vi "CCSA RPJ SLJC PF SubVI009.vi"(2 "Patrón original":T1, 3 "Toma original":T1) -> (0 "Toma original":T1(plugin-control), 1 "Patrón corregido":T1(plugin-control))   [LabVIEW 2021]
doc: "Traslada el patrón a la misma posición que la toma de la cámara para empalmar sus contornos"
uses:
  <vilib>/vision/Image Controls.llb/IMAQ Image.ctl
panel:
  out "Patrón original":T1(plugin-control)
  out "Centroide Patron":cluster{"X Centroid":sgl, "Y Centroid":sgl}
  out "Centroide Captura":cluster{"X Centroid":sgl, "Y Centroid":sgl}
  # "CUEVAS CERÓN SERGIO ALBERTO\nREYES PÉREZ JAVIER\nSALCEDO LICEA JUAN CARLOS"
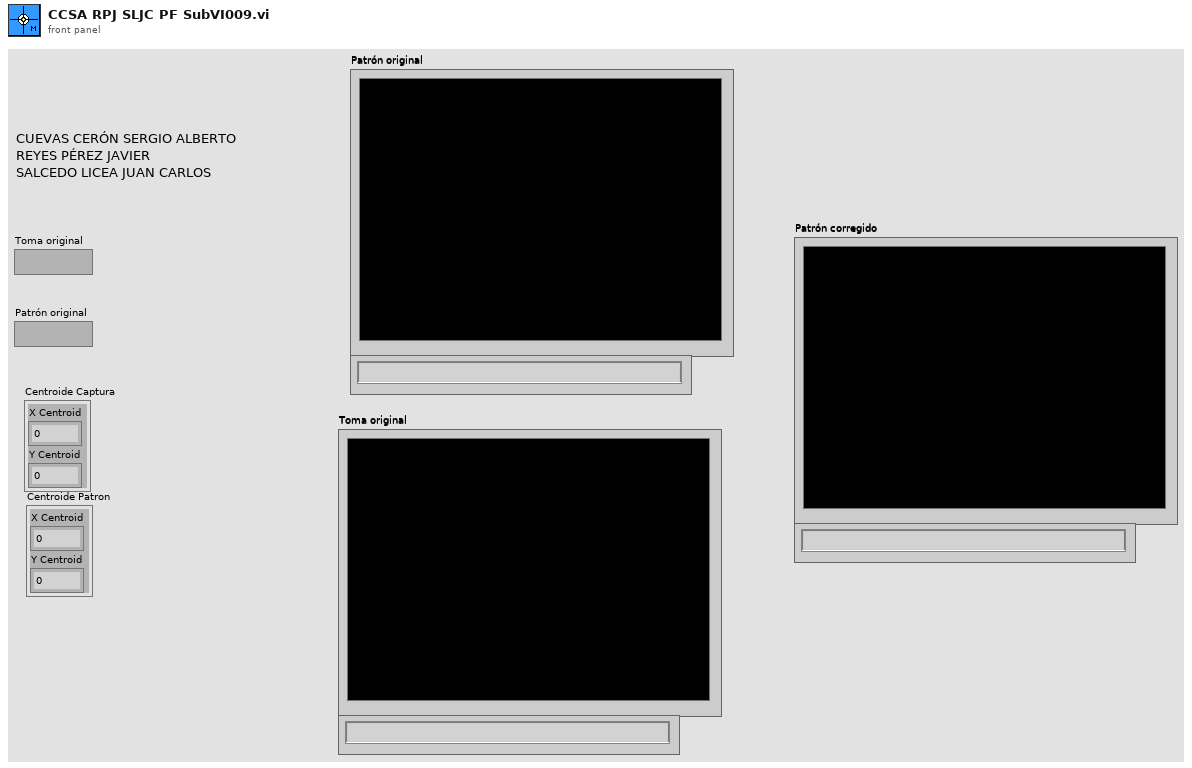
[diagram p1: front panel]
types:
  T1 = typedef "IMAQ Image.ctl" = refnum<image>
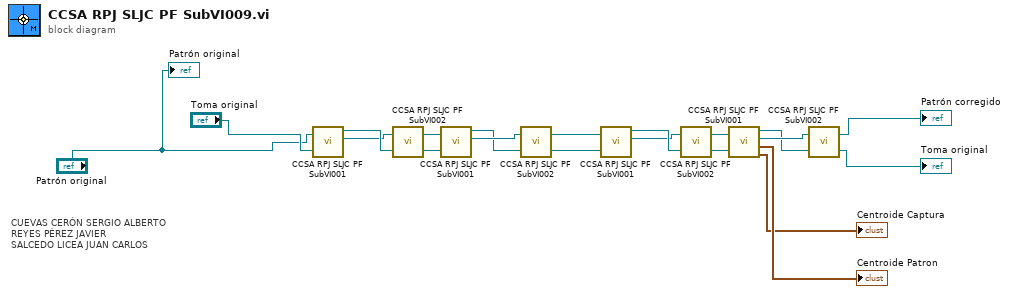
[diagram p0: block diagram]
diagram:
  # "CUEVAS CERÓN SERGIO ALBERTO\nREYES PÉREZ JAVIER\nSALCEDO LICEA JUAN CARLOS"
  n1 = call "CCSA RPJ SLJC PF SubVI001.vi"("Patrón original"="Patrón original", "Toma original"="Toma original") -> ("Patron trasladada"=w18:T1, "Toma original(dup)"=w17:T1)  [unwired: 2 out]
  n2 = call "CCSA RPJ SLJC PF SubVI002.vi"("Patrón original"=w18, "Toma original"=w17) -> ("Toma original"=w15:T1, "Patron rotado"=w16:T1)
  n3 = call "CCSA RPJ SLJC PF SubVI001.vi"("Patrón original"=w16, "Toma original"=w15) -> ("Patron trasladada"=w13:T1, "Toma original(dup)"=w14:T1)  [unwired: 2 out]
  n4 = call "CCSA RPJ SLJC PF SubVI002.vi"("Patrón original"=w13, "Toma original"=w14) -> ("Toma original"=w5:T1, "Patron rotado"=w6:T1)
  n5 = call "CCSA RPJ SLJC PF SubVI001.vi"("Patrón original"=w6, "Toma original"=w5) -> ("Patron trasladada"=w12:T1, "Toma original(dup)"=w11:T1)  [unwired: 2 out]
  n6 = call "CCSA RPJ SLJC PF SubVI002.vi"("Patrón original"=w12, "Toma original"=w11) -> ("Toma original"=w9:T1, "Patron rotado"=w10:T1)
  n7 = call "CCSA RPJ SLJC PF SubVI001.vi"("Patrón original"=w10, "Toma original"=w9) -> ("Patron trasladada"=w7:T1, "Toma original(dup)"=w8:T1, "Centroide patron trasladado"=→"Centroide Patron":cluster{"X Centroid":sgl, "Y Centroid":sgl}, "Centroide toma original"=→"Centroide Captura":cluster{"X Centroid":sgl, "Y Centroid":sgl})
  n8 = call "CCSA RPJ SLJC PF SubVI002.vi"("Patrón original"=w7, "Toma original"=w8) -> ("Toma original"=→"Toma original":T1, "Patron rotado"=→"Patrón corregido":T1)
  "Patrón original" <- "Patrón original"
